vi "Read Multi Eval Meas Modulation Results.vi"(8 "error in (no error)":errorcluster, 9 "Result Type (Current)":i32(ring) items=["Current", "Average", "Extreme", "Standard Deviation"], 10 "Instance (1)":T1=1, 11 "VISA resource name":refnum<visa-resource-name>) -> (0 "error out":errorcluster, 1 "Modulation Results":dbl[](array[numeric]) format="%^.3e", 2 "Reliability":i32, 3 "VISA resource name out":refnum<visa-resource-name>)   [LabVIEW 2015, in "Rohde&Schwarz CMXP NR FR2 Measurement.lvlib"]
doc: "Starts a new single shot measurement and returns the multi eval measurement modulation values.\n\nAttributes:\nRSCMXPNRFR2M_ATTR_READ_MULTI_EVAL_MEASUREMENT_MODULATION_AVERAGE_RESULTS\nRSCMXPNRFR2M_ATTR_READ_MULTI_EVAL_MEASUREMENT_MODULATION_CURRENT_RESULTS\nRSCMXPNRFR2M_ATTR_READ_MULTI_EVAL_MEASUREMENT_MODULATION_EXTREME_RESULTS\nRSCMXPNRFR2M_ATTR_READ_MULTI_EVAL_MEASUREMENT_MODULATION_STANDARD_DEVIATION_RESULTS\n\nRemote-control commands:\nREAD:NRMMw:MEAS<i>:MEValuation:MODulation:AVERage?\nREAD:NRMMw:MEAS<i>:MEValuation:MODulation:CURRent?\nREAD:NRMMw:MEAS<i>:MEValuation:MODulation:EXTReme?\nREAD:NRMMw:MEAS<i>:MEValuation:MODulation:SDEViation?"
uses:
  <instrlib>/Rohde&Schwarz CMXP NR FR2 Measurement/Rohde&Schwarz CMXP NR FR2 Measurement.lvlib
  <instrlib>/Rohde&Schwarz CMXP NR FR2 Measurement/Private/_Instance.ctl
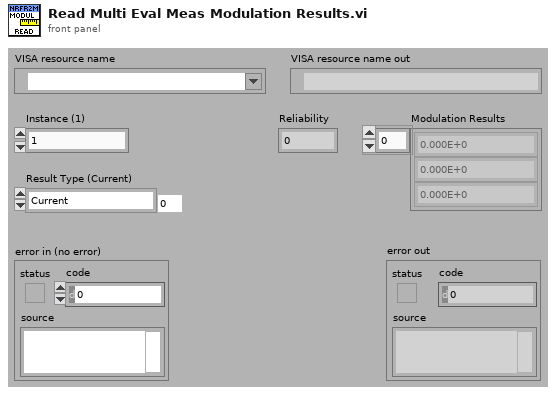
[diagram p1: front panel]
types:
  T1 = typedef "Rohde&Schwarz CMXP NR FR2 Measurement.lvlib/_Instance.ctl" = i32
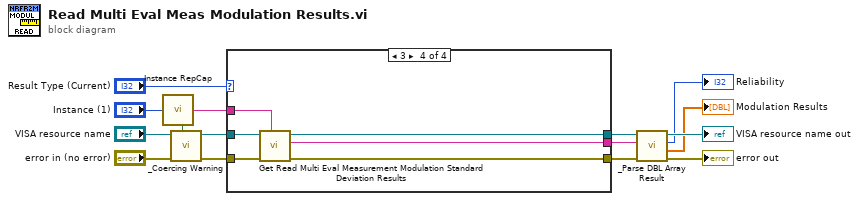
[diagram p0: block diagram]
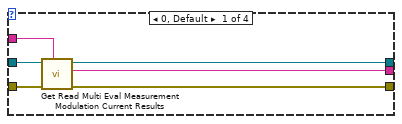
[diagram p2: hidden frame]
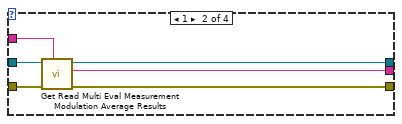
[diagram p3: hidden frame]
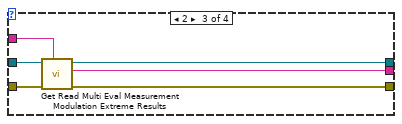
[diagram p4: hidden frame]
diagram:
  n1 = call <instrlib>:"Instance RepCap.vi"("Instance In"="Instance (1)") -> ("In Range?"=w4:bool, "RepCap Identifier Out"=w15:string)  [unwired: 1 in]
  n2 = call <instrlib>:"_Coercing Warning.vi"("In Range?"=w4, "error in (no error)"="error in (no error)", "VISA resource name"="VISA resource name") -> ("error out"=w2:errorcluster, "VISA resource name out"=w3:refnum<visa-resource-name>)  [unwired: 7 in]
  n3 = case shown="3" "Result Type (Current)" {
    tunnel: w15 -> [w21 w27 w33 w39]
    tunnel: w2 -> [w20 w26 w32 w38]
    tunnel: w3 -> [w19 w25 w31 w37]
    tunnel: [w18 w24 w30 w36] -> w14
    tunnel: [w17 w23 w29 w35] -> w13
    tunnel: [w16 w22 w28 w34] -> w8
    frame 0, Default {
      n4 = call "Get Read Multi Eval Measurement Modulation Current Results"("Repeated Capabilities"=w21, "error in (no error)"=w20, "instrument handle"=w19) -> ("error out"=w18:errorcluster, "Read Multi Eval Measurement Modulation Current Results"=w16:string, "instrument handle out"=w17:refnum<visa-resource-name>)  [unwired: 6 in]
    }
    frame 1 {
      n5 = call "Get Read Multi Eval Measurement Modulation Average Results"("Repeated Capabilities"=w27, "error in (no error)"=w26, "instrument handle"=w25) -> ("error out"=w24:errorcluster, "Read Multi Eval Measurement Modulation Average Results"=w22:string, "instrument handle out"=w23:refnum<visa-resource-name>)  [unwired: 6 in]
    }
    frame 2 {
      n6 = call "Get Read Multi Eval Measurement Modulation Extreme Results"("Repeated Capabilities"=w33, "error in (no error)"=w32, "instrument handle"=w31) -> ("error out"=w30:errorcluster, "Read Multi Eval Measurement Modulation Extreme Results"=w28:string, "instrument handle out"=w29:refnum<visa-resource-name>)  [unwired: 6 in]
    }
    frame 3 {
      n7 = call "Get Read Multi Eval Measurement Modulation Standard Deviation Results"("Repeated Capabilities"=w39, "error in (no error)"=w38, "instrument handle"=w37) -> ("error out"=w36:errorcluster, "Read Multi Eval Measurement Modulation Standard Deviation Results"=w34:string, "instrument handle out"=w35:refnum<visa-resource-name>)  [unwired: 6 in]
    }
  }
  n8 = call <instrlib>:"_Parse DBL Array Result.vi"("error in (no error)"=w14, "Input String"=w8, "VISA resource name"=w13) -> ("error out"=→"error out":errorcluster, "Results"=→"Modulation Results":dbl[], "Reliability"=→"Reliability":i32, "VISA resource name out"=→"VISA resource name out":refnum<visa-resource-name>)  [unwired: 5 in]
